vi "Get Document Dir.vi"() -> (0 "document dir":path)   [LabVIEW 2013]
uses:
  <vilib>/Utility/sysdir.llb/System Directory Type.ctl
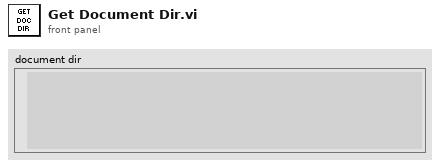
[diagram p1: front panel]
types:
  T1 = typedef "System Directory Type.ctl" = i32
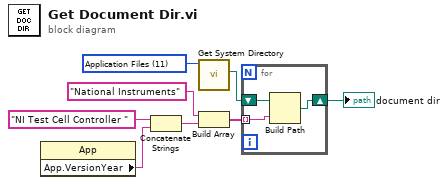
[diagram p0: block diagram]
diagram:
  w8 = T1 11 items=["User Home"=0, "User Desktop"=1, "User Documents"=2, "User Application Data"=3, "User Preferences"=4, "User Temporary"=5, "Public Documents"=6, "Public Application Data"=7, "Public Preferences"=8, "Public Cache"=13, "System Core Libraries"=9, "System Installed Libraries"=10, "Application Files"=11, "Boot Volume Root"=12] ("system directory type")
  n1 = property class="App"() -> ("App.VersionYear"=w5:string)  [unwired: 2 in, 2 out]
  n2 = Concatenate Strings("NI Test Cell Controller ", w5) -> (w2:string)
  n3 = call <vilib>:"Get System Directory.vi"("system directory type"=w8) -> ("system directory"=w7:path)  [unwired: 10 in]
  n4 = Build Array("National Instruments", w2) -> (w1:string[])
  n5 = for {
    tunnel: w1 -> [w9] mode=indexing
    shift-right: [w10] -> w6
    shift-left: w7 -> [w11]
    n6 = Build Path(base path=w11, name or relative path=w9) -> (appended path=w10:path)
  }
  "document dir" <- w6
